vi "strain-data-buffer.vi"(7 "cmd":enum16{"clear", "add", "read"}(ring), 11 "History Data":waveform(dbl)[](array[waveform])) -> (3 "data out":waveform(dbl)[][](array[waveform]))   [LabVIEW 2013]
panel:
  out "크기":i32[](array[numeric])
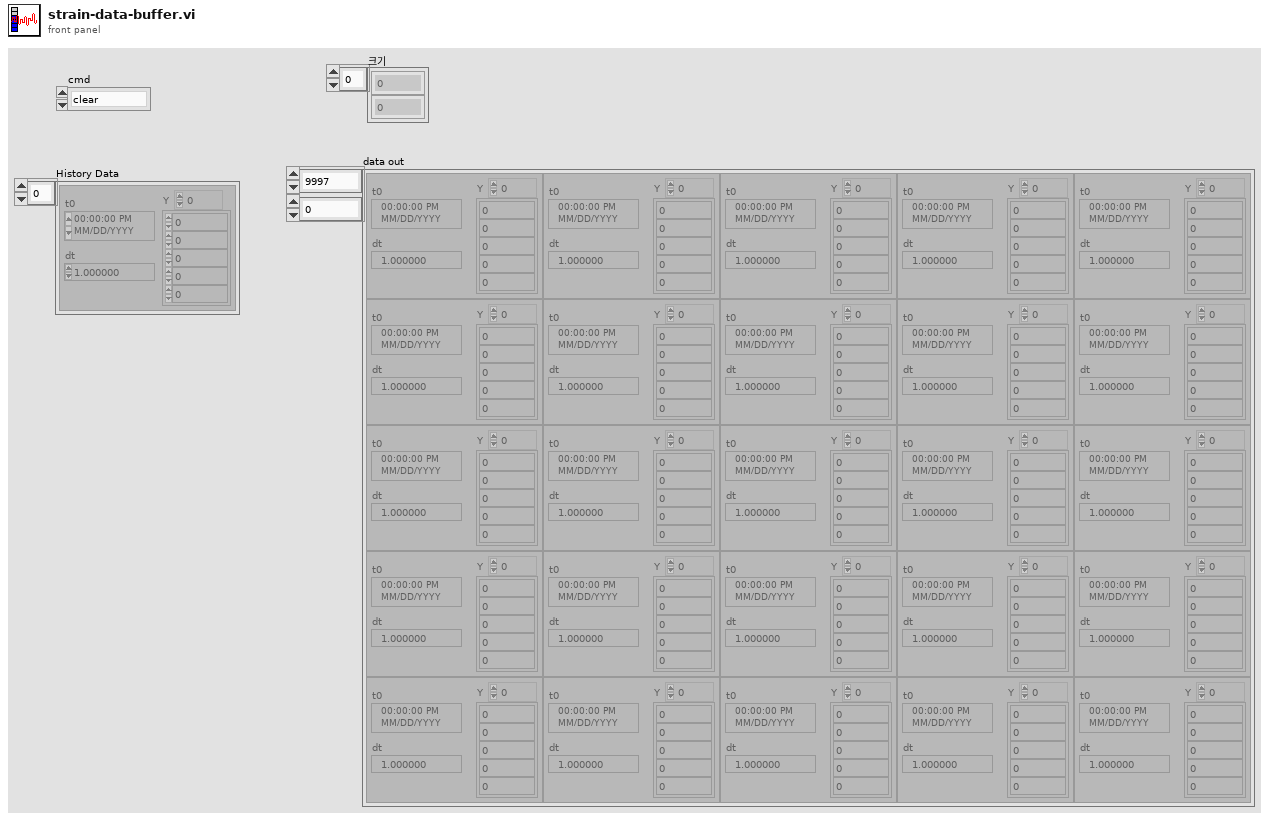
[diagram p1: front panel]
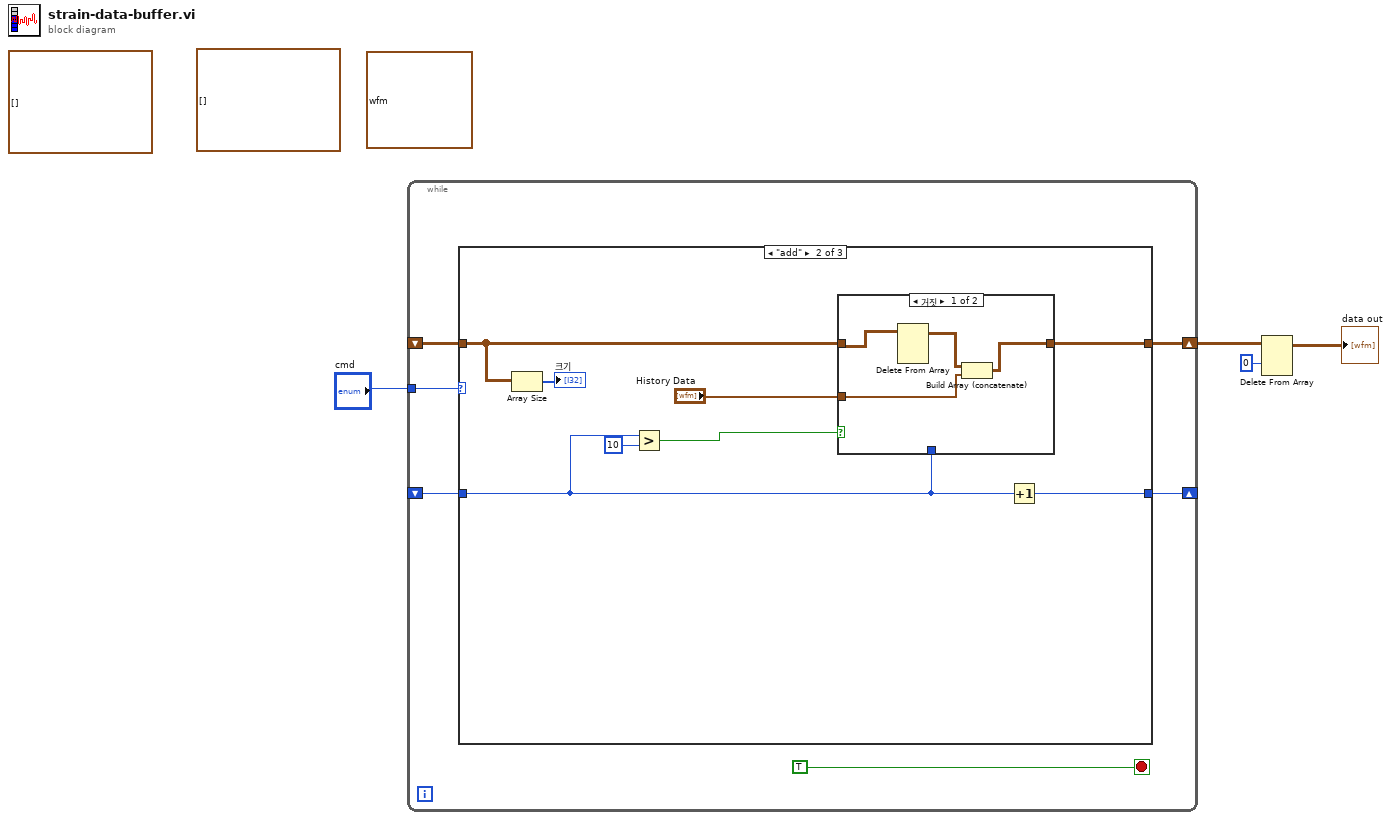
[diagram p0: block diagram]
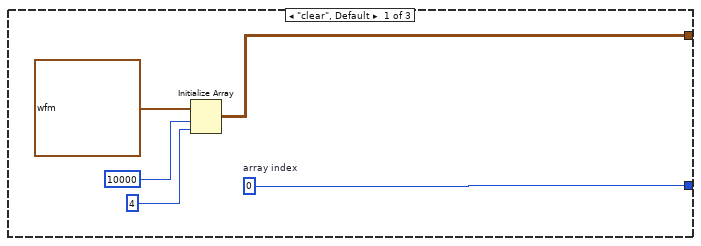
[diagram p2: hidden frame]
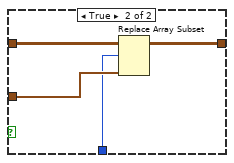
[diagram p3: hidden frame]
diagram:
  (unwired) waveform(dbl)[][] [] ("히스토리 데이터")
  (unwired) waveform(dbl) {"t0"=timestamp(0 s since 1904-01-01), "dt"=1.0, "Y"=[]}
  (unwired) waveform(dbl)[] [] ("History Data")
  n1 = while {
    tunnel: "cmd" -> [w9]
    shift-right: [w7] -> w3
    shift-left: _ -> [w8]
    shift-right: [w6] -> _
    shift-left: _ -> [w5]
    stop <- TRUE stop-if-true
    n2 = case shown="\"add\"" w9 {
      tunnel: w8 -> [_ w20 w33]
      tunnel: [w12 w23 w33] -> w7
      tunnel: [w13 w22 w32] -> w6
      tunnel: w5 -> [_ w18 w32]
      frame "clear", Default {
        w13 = 0  # array index
        n3 = Initialize Array(waveform(dbl) {"t0"=timestamp(0 s since 1904-01-01), "dt"=0.00062, "Y"=[]}, 10000 ("차원 크기"), 4 ("차원 크기")) -> (w12:waveform(dbl)[][])
      }
      frame "add" {
        n4 = Array Size(array=w20) -> (size(s)=→"크기":i32[])
        n5 = Greater?(x=w18, y=10) -> (0:w16:bool)
        n6 = case shown="거짓" w16 {
          tunnel: [w24 w31] -> w23
          tunnel: "History Data" -> [w25 w30]
          tunnel: w20 -> [w27 w29]
          tunnel: w18 -> [_ w28]
          frame False {
            n7 = Delete From Array(array=w27) -> (array with subset deleted=w26:waveform(dbl)[][])  [unwired: 3 in, 1 out]
            n8 = Build Array (concatenate)(w26, w25) -> (w24:waveform(dbl)[][])
          }
          frame True {
            n9 = Replace Array Subset(array=w29, new element=w30, index (row)=w28) -> (w31:waveform(dbl)[][])  [unwired: 1 in]
          }
        }
        n10 = Increment(x=w18) -> (x+1=w22:i32)
      }
      frame "read" {
      }
    }
  }
  n11 = Delete From Array(array=w3, index (row)=0 ("인덱스 (행)")) -> (array with subset deleted=→"data out":waveform(dbl)[][])  [unwired: 2 in, 1 out]
